vi "Sample--Conti.vi"() -> ()   [LabVIEW 2013]
doc: "This samples demonstrates how to sample continuous waveform."
uses:
  <userlib>/ArtScope/Trigger/ArtScope_ConfigureTriggerSoftWare.vi
  <userlib>/ArtScope/Fetch/ArtScope_FetchVoltage.vi
  <userlib>/ArtScope/_SubVI/ArtScope_ArrayByChannel_DBL.vi
panel:
  in  "reference position":dbl
  in  "num samples":i32=1000
  in  "range(Vpp)":i32(ring) items=["20V", "10V", "2V", "40V", "16V", "8V", "4V", "1.6V", "800m", "400m", "160m", "80m", "40m"]
  in  "offset(mV)":i32
  in  "Stop":bool
  out "waveform":dbl[][](graph)
  out "ErrorOutput":errorcluster
  in  "min record length":i32=1000
  in  "min sample rate":dbl=8000000.0
  in  "coupling":i32(ring) items=["DC", "AC"]
  in  "channel name":string="0,1"
  in  "resource name":string="Dev1"
  # "Vertical"
  # "Horizontal"
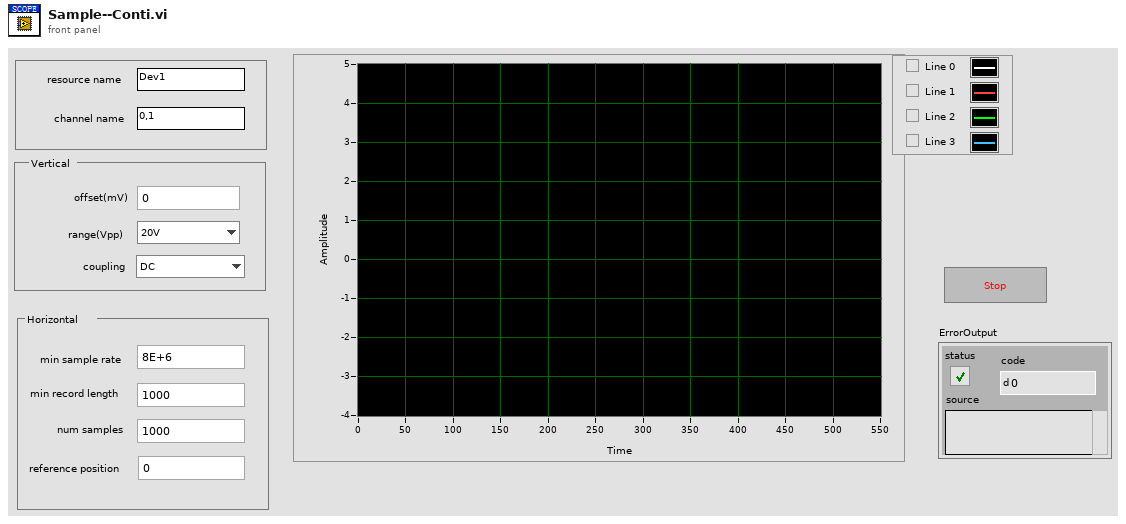
[diagram p1: front panel]
types:
  T1 = cluster{"fLSB":cluster{dbl, dbl, dbl, dbl, dbl, dbl, dbl, dbl}, "RangeValue":cluster{dbl, dbl, dbl, dbl, dbl, dbl, dbl, dbl}, "wMaxLSB":u32, "TriggerMode":i32, "sampLengthPerChan":u32, "pAvailSampsPoints":u32, "channelCount":i32}
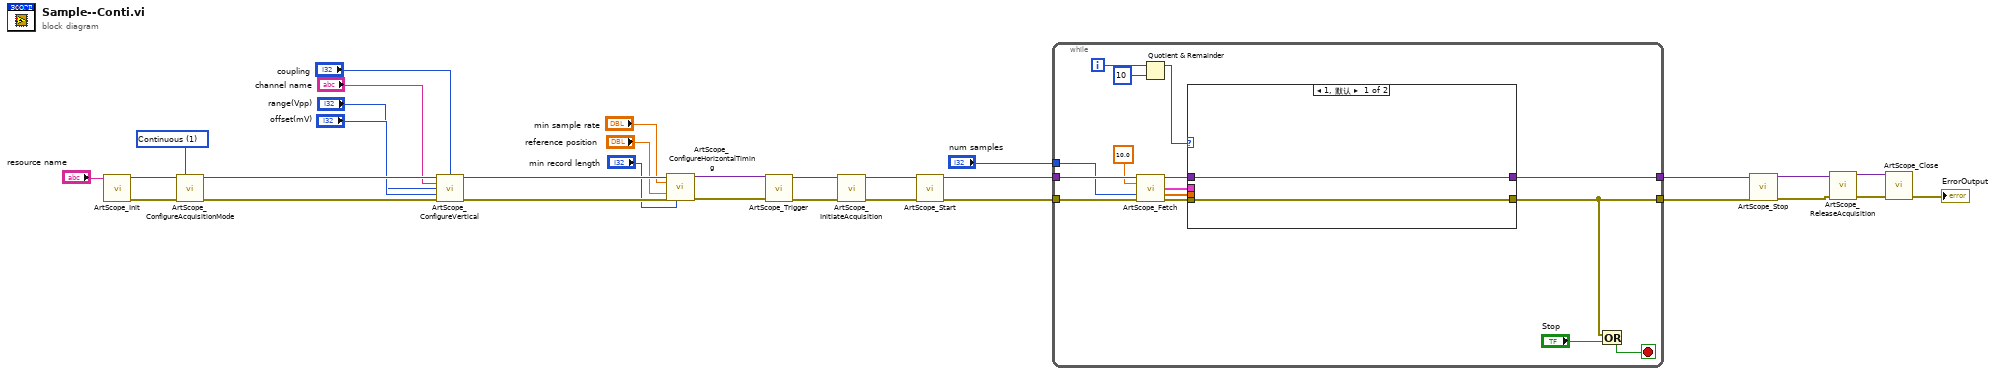
[diagram p0: block diagram]
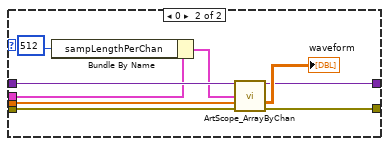
[diagram p2: hidden frame]
diagram:
  w28 = 1 items=["Finite", "Continuous"] ("AcuqMode")
  n1 = call <userlib>:"ArtScope_Init.vi"("task name"="resource name") -> ("task handle"=w31:variant, "error out"=w30:errorcluster)  [unwired: 13 in]
  n2 = call <userlib>:"ArtScope_ConfigureAcquisitionMode.vi"("task handle"=w31, "acquisition mode"=w28, "error in (no error)"=w30) -> ("task handle"=w27:variant, "error out"=w26:errorcluster)  [unwired: 11 in]
  n3 = call <userlib>:"ArtScope_ConfigureVertical.vi"("task handle"=w27, "coupling"="coupling", "channels"="channel name", "range(Vpp)"="range(Vpp)", "offset"="offset(mV)", "error in (no error)"=w26) -> ("task handle"=w24:variant, "error out"=w23:errorcluster)  [unwired: 8 in]
  n4 = call <userlib>:"ArtScope_ConfigureHorizontalTiming.vi"("task handle"=w24, "min sample rate"="min sample rate", "reference position"="reference position", "error in (no error)"=w23, "min record length"="min record length") -> ("task handle"=w21:variant, "error out"=w20:errorcluster)  [unwired: 9 in]
  n5 = call-poly <userlib>:"ArtScope_Trigger.vi"("task handle"=w21, "error in (no error)"=w20) -> ("task handle"=w16:variant, "error out"=w15:errorcluster)  [unwired: 12 in]
  n6 = call <userlib>:"ArtScope_InitiateAcquisition.vi"("task handle"=w16, "error in (no error)"=w15) -> ("task handle"=w13:variant, "error out"=w14:errorcluster)  [unwired: 12 in]
  n7 = call <userlib>:"ArtScope_Start.vi"("task handle"=w13, "error in (no error)"=w14) -> ("task handle"=w8:variant, "error out"=w7:errorcluster)  [unwired: 12 in]
  n8 = while {
    tunnel: w8 -> [w46]
    tunnel: w7 -> [w45]
    tunnel: [w36] -> w6
    tunnel: [w33] -> w5
    tunnel: "num samples" -> [w39]
    i -> [w43]
    stop <- w40 stop-if-true
    n9 = call-poly <userlib>:"ArtScope_Fetch.vi"("task handle"=w46, "timeout"=10.0 ("Timeout"), "num samples"=w39, "error in (no error)"=w45) -> ("task handle"=w38:variant, "wfm info"=w34:T1, "data"=w35:dbl[], "error out"=w37:errorcluster)  [unwired: 8 in]
    n10 = Quotient & Remainder(x=w43, y=10) -> (x-y*floor(x/y)=w32:i32)  [unwired: 1 out]
    n11 = case shown="1, 默认" w32 {
      tunnel: w38 -> [w48 w57]
      tunnel: w37 -> [w47 w56]
      tunnel: [w47 w55] -> w36
      tunnel: w35 -> [_ w54]
      tunnel: w34 -> [_ w53]
      tunnel: [w48 w49] -> w33
      frame 1, Default {
      }
      frame 0 {
        n12 = Bundle By Name(cluster=w53, "sampLengthPerChan"=u32 512 ("FetchLength")) -> (w51:T1)
        n13 = call-poly <userlib>:"ArtScope_ArrayByChan.vi"("task handle"=w57, "wfm info"=w51, "1D data"=w54, "error in (no error)"=w56) -> ("task handle"=w49:variant, "2D data"=→"waveform":dbl[][], "error out"=w55:errorcluster)  [unwired: 9 in]
      }
    }
    n14 = Or(x=w36, y="Stop") -> (x .or. y?=w40:bool)
  }
  n15 = call <userlib>:"ArtScope_Stop.vi"("task handle"=w5, "error in (no error)"=w6) -> ("task handle"=w9:variant, "error out"=w10:errorcluster)  [unwired: 12 in]
  n16 = call <userlib>:"ArtScope_ReleaseAcquisition.vi"("task handle"=w9, "error in (no error)"=w10) -> ("task handle"=w11:variant, "error out"=w12:errorcluster)  [unwired: 12 in]
  n17 = call <userlib>:"ArtScope_Close.vi"("task handle"=w11, "error in (no error)"=w12) -> ("error out"=→"ErrorOutput":errorcluster)  [unwired: 13 in]
